vi "SimpleMotorFeedForward_Example_2.vi"() -> ()   [LabVIEW 2019]
uses:
  <vilib>/Rock Robotics/WPI/ThirdParty/JAS_Junk/TrajLib/LinearFilter_ResetToValue.vi
  <vilib>/Rock Robotics/WPI/ThirdParty/JAS_Junk/TrajLib/LinearFilter_Calculate.vi
  <vilib>/Rock Robotics/WPI/ThirdParty/JAS_Junk/TrajLib/SimpleMotorFF_Calculate.vi
  <vilib>/Rock Robotics/WPI/ThirdParty/JAS_Junk/TrajLib/LinearFilter_MovingAverage.vi
  <vilib>/Rock Robotics/WPI/ThirdParty/JAS_Junk/TrajLib/LinearFilter_LowPassBW1.vi
  <vilib>/Rock Robotics/WPI/ThirdParty/JAS_Junk/TrajLib/LinearFilter_LowPassBW2.vi
  <vilib>/Rock Robotics/WPI/ThirdParty/JAS_Junk/TrajLib/LinearFilter_HighPassBW1.vi
  <vilib>/Rock Robotics/WPI/ThirdParty/JAS_Junk/TrajLib/LinearFilter_HighPassBW2.vi
  <vilib>/Rock Robotics/WPI/ThirdParty/JAS_Junk/TrajLib/Trajectory_Library.lvlib
panel:
  in  "Tab Control":T1(tab)
  out "Running Ka AutoTune":bool
  in  "Execute Ka AutoTune":bool
  out "Filtered Setpoint \nRate of Change":dbl format="%11.3f"
  in  "Auto Setpoint":bool
  out "CO Trend":dbl(graph)
  out "SP, PV Trend":T2(graph)
  in  "Desired Speed":dbl(slide)=-0.22222222222222499 scale=-10.0..10.0 scale format="%#.1f"
  in  "Enable Noise":bool
  in  "Ks":dbl format="%#_13g"
  in  "Kv":dbl=0.1 format="%#_13g"
  in  "Ka":dbl format="%#_13g"
  out "Motor Dmd":dbl format="%13.3f"
  out "Filtered Speed":dbl format="%12.2f"
  out "Filtered Speed \nError":dbl format="%11.3f"
  in  "Ka Testing Parameters":T3={"Min SP"=0.0, "Max SP"=9.0, "Min Eval SP"=1.5, "Max Eval SP"=7.5, "Ramp Rate"=0.66}
  out "Test Complete":bool
  out "Ka Calc":dbl=-1.0 format="%#_8g"
  out "Ka StdDev":dbl=-1.0 format="%#_8g"
  out "Error":bool
  # "Simple Motor Feedforward Example 2"
  # "FT/SEC"
  # "FT/SEC"
  # "Sample procedure to tune Simple Motor Feedforward Ks, Kv, Ka.\n\nThis is just one possible method to do the tuning.  Other methods, including using the characterization tool, can be used.\n\n1) Set the Ka and Ks to 0.0.   Set Kv to be 1 / Estimated Maximum Speed.   (For many robots 10 feet/sec works as a starting point).\n     If using any closed loop control, such as a PID, disable the closed loop control, either by removing the code, or for the advanced\n    PID, putting it in manual mode.  (This simulation does not have a closed loop controller.)\n\n2)  Set the motor output at a small value.  (Example 0.15).  To do this set the speed demand to a small value, such as 1.5 Ft/Sec.\n      After the robot comes to constant speed, record the Motor Demand CO and Actual Speed (PV)\n\n3) Set the motor output to a large value (Example 0.90).   To do this, set the speed demand to a large value, such as 9.0 Ft/Sec\n     After the robot (or this simulation) comes to a constant speed, record the Motor Demand (CO) and the Actual Speed (PV).\n\n4) Ks and Kv can be calculated from the straight line equation:\n                               Motor Dmd CO = Sign( Speed_Setpoint) x Ks + Speed_Setpoint x Kv\n                                          Sign = 1 when Speed_Setoint > 0.0, \n                                          0 when Speed_Setpoint = 0 and, \n                                          -1 when Speed_Setpoint < 0\n\n5) The Ka term represents the additional Motor Demand CO needed to cancel the lag of the motor.   Technically, the Ka term\n      represents a \"lead\" function (sometimes referred to as a kicker circuit).  The amount that Ka adds to the Motor Demand CO\n      is  Ka x Speed_Setpoint Rate of Change (units/second).  Therefore, while the speed is ramping, one knows, or can be\n      calculated:   \n                             - Setpoint Rate of Change\n                             - Speed, speed setpoint, motor demand a time \"n\"\n                             - motor demand at time \"m\" where speed_m = speed_setpoint_n\n  \n    This should be enough data to calculate a value for Ka:\n                              Ka = (motor_demand_m - motor_demand_n ) / setpoint_rate_of_change\n\n     The Ka term will cause the speed to overshoot slightly during a ramp.  This is an expected side-affect of this type of \n     algorithm.  \n\n6) Test everything and look at the trend to ensure the response is acceptable.    Adjust as desired."
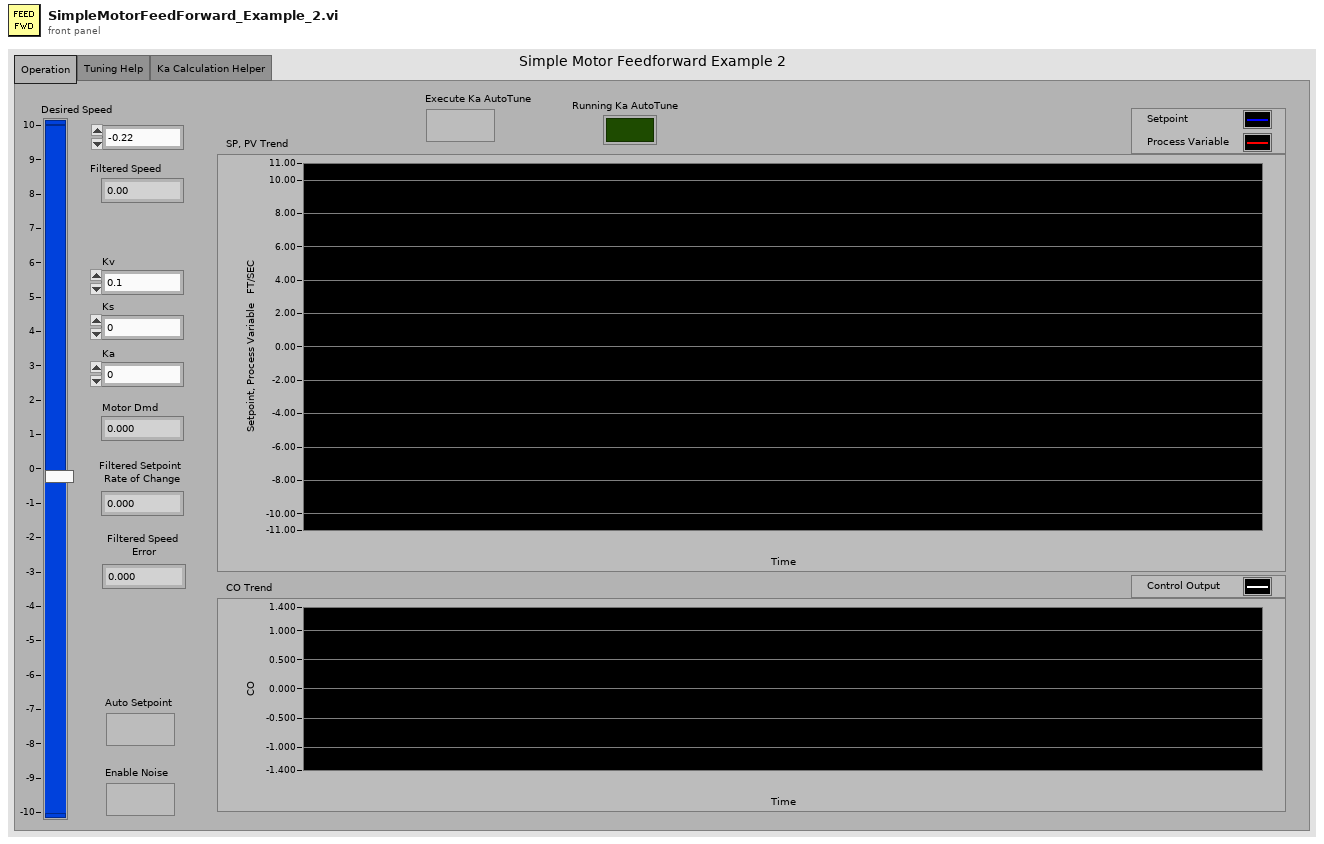
[diagram p1: front panel]
types:
  T1 = enum32{"Operation", "Tuning Help", "Ka Calculation Helper"}
  T2 = cluster{"SpeedSetpoint":dbl, "LeftWheelSpeed":dbl}
  T3 = cluster{"Min SP":dbl, "Max SP":dbl, "Min Eval SP":dbl, "Max Eval SP":dbl, "Ramp Rate":dbl}
  T4 = enum16{"Moving Average", "Low Pass 1st Order Butterworth", "Low Pass 2nd Order Butterworth", "High Pass 1st Order Butterworth", "High Pass 2nd Order Butterworth"}
  T5 = typedef "Trajectory_Library.lvlib/SIMPLE_MOTOR_FF.ctl" = cluster{"Ks":dbl, "Kv":dbl, "Ka":dbl, "KnInv":dbl}
  T6 = cluster{"Speed Setpoint Ft/Sec":dbl, "Motor Speed":dbl}
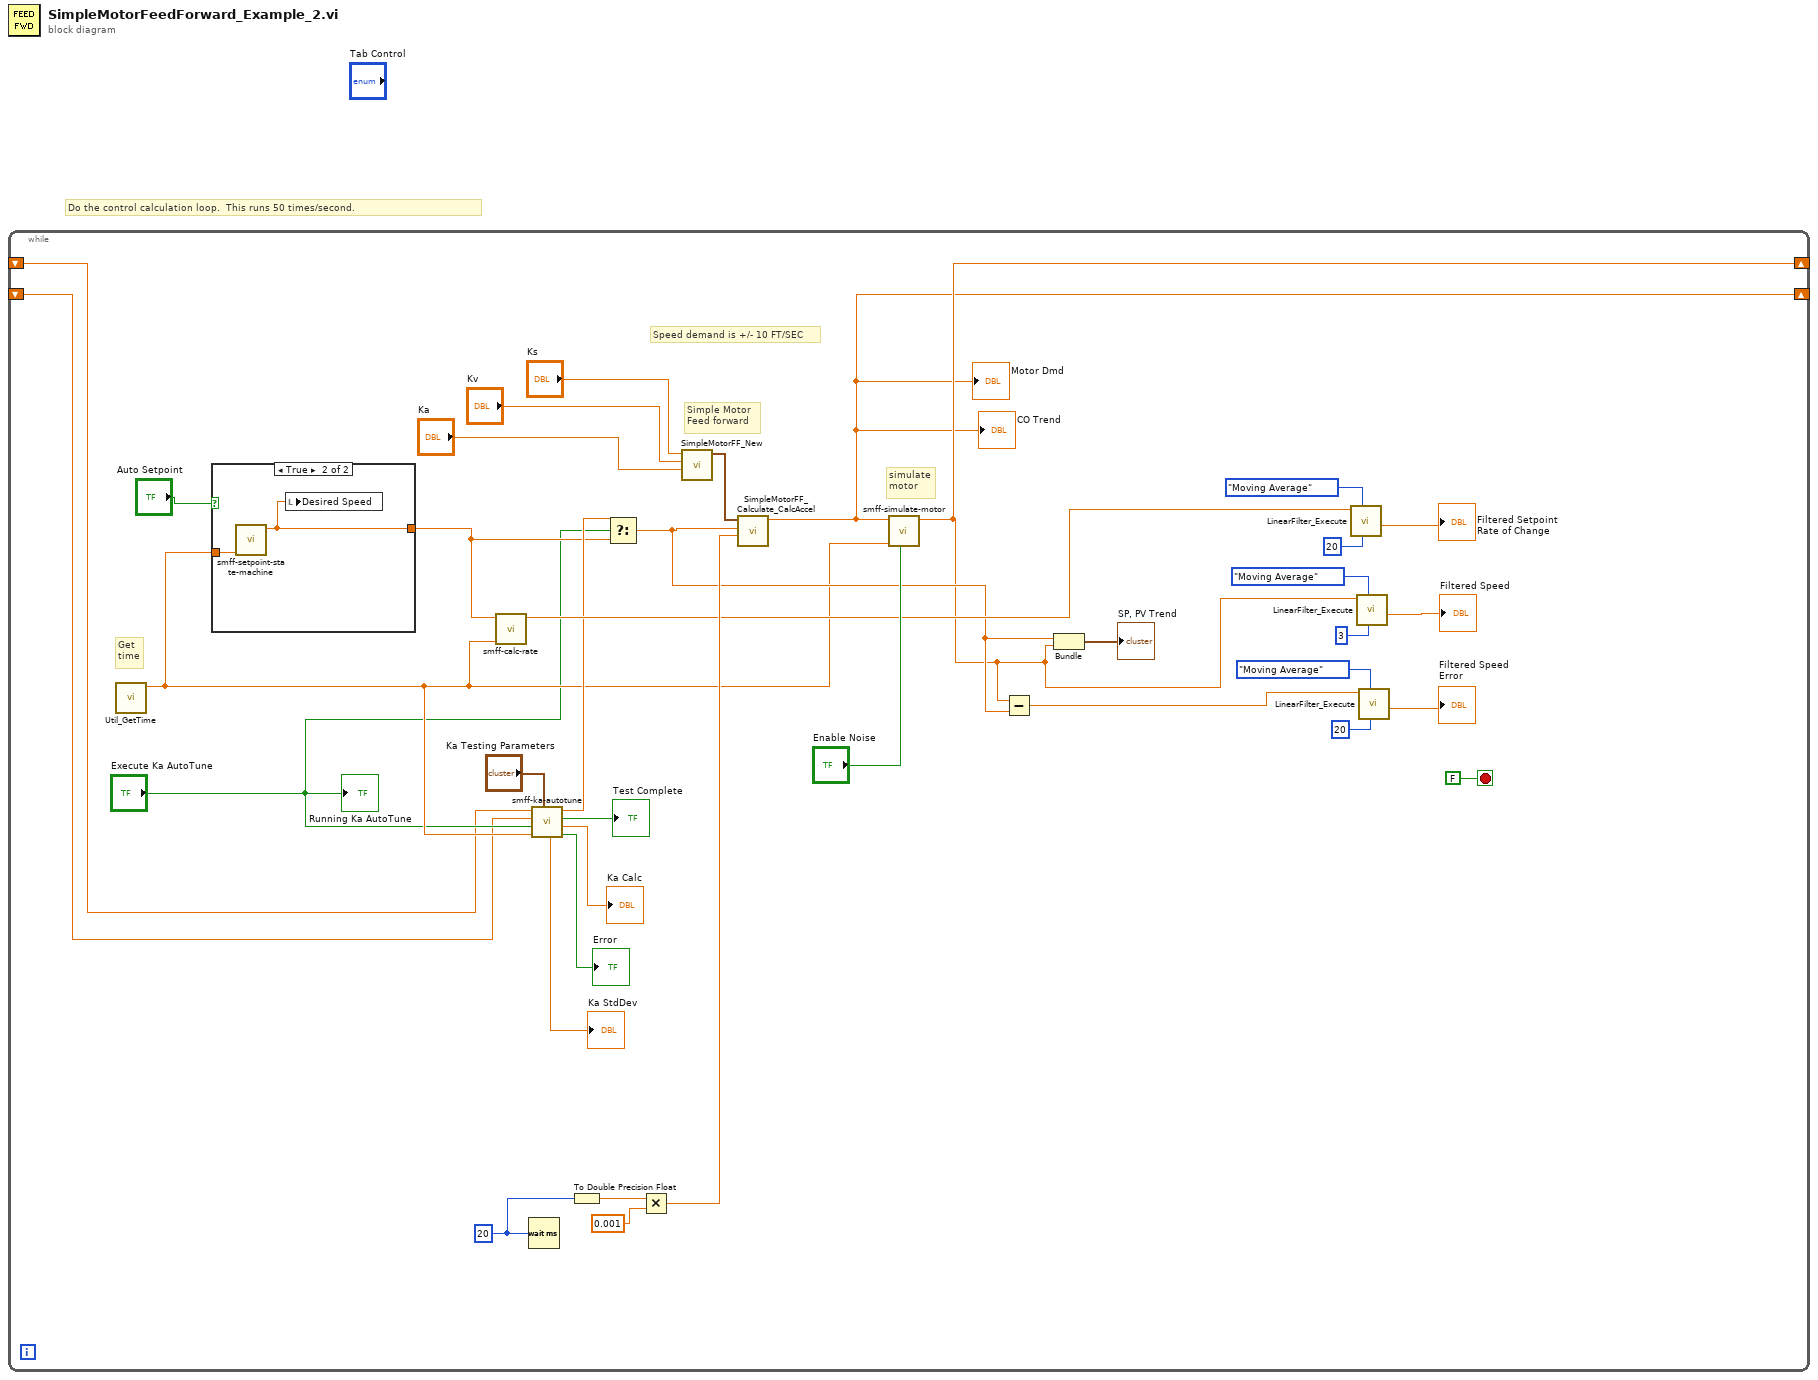
[diagram p0: block diagram]
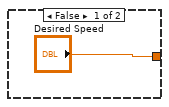
[diagram p2: hidden frame]
diagram:
  # "Do the control calculation loop.  This runs 50 times/second."
  n1 = while {
    shift-right: [w6] -> _
    shift-left: _ -> [w4]
    shift-right: [w5] -> _
    shift-left: _ -> [w3]
    stop <- FALSE stop-if-true
    w36 = u32 20 ("milliseconds to wait")
    # "Get\ntime"
    # "Speed demand is +/- 10 FT/SEC"
    # "simulate\nmotor"
    # "Simple Motor\nFeed forward"
    n2 = call <vilib>:"Util_GetTime.vi"() -> ("FPGA_Time_Seconds"=w8:dbl)  [unwired: 10 in, 1 out]
    n3 = case shown="True" "Auto Setpoint" {
      tunnel: w8 -> [_ w40]
      tunnel: ["Desired Speed" w39] -> w12
      frame False {
      }
      frame True {
        n4 = call "smff-setpoint-state-machine.vi"("Time pass through"=w40) -> ("Speed Setpoint Ft/Sec"=w39:dbl)  [unwired: 9 in, 1 out]
        n5 = local write "Desired Speed"(w39) -> ()
      }
    }
    n6 = call "smff-calc-rate.vi"("Time pass through"=w8, "Value"=w12) -> ("Value Rate"=w15:dbl)  [unwired: 9 in]
    n7 = Wait (ms)(milliseconds to wait=w36) -> ()  [unwired: 1 out]
    n8 = call "smff-ka-autotune.vi"("SimpleMotorFeedforward_KaTune_Pack"="Ka Testing Parameters", "PassThroughTime"=w8, "Run Test"="Execute Ka AutoTune", "ControlOutput CO"=w3, "ProcVariable PV"=w4) -> ("Error"=→"Error":bool, "Ka Calc"=→"Ka Calc":dbl, "Test Complete"=→"Test Complete":bool, "SetPoint"=w13:dbl, "Ka StdDev"=→"Ka StdDev":dbl)  [unwired: 2 out]
    n9 = To Double Precision Float(number=w36) -> (double precision float=w30:dbl)
    n10 = Select(t=w13, s="Execute Ka AutoTune", f=w12) -> (s? t:f=w14:dbl)
    n11 = Multiply(x=w30, y=0.001) -> (x*y=w28:dbl)
    n12 = call <vilib>:"SimpleMotorFF_New.vi"("Ka"="Ka", "Kv"="Kv", "Ks"="Ks") -> ("SIMPLE_MOTOR_FF"=w34:T5)  [unwired: 8 in]
    n13 = call <vilib>:"SimpleMotorFF_Calculate_CalcAccel.vi"("dT_Sec"=w28, "VelSp"=w14, "SIMPLE_MOTOR_FF"=w34) -> ("FeedForward"=w5:dbl)  [unwired: 8 in]
    "Motor Dmd" <- w5
    "CO Trend" <- w5
    n14 = call "smff-simulate-motor.vi"("Use Noise"="Enable Noise", "Time"=w8, "CO-ControlOutput"=w5) -> ("Motor Speed"=w6:dbl)  [unwired: 8 in]
    n15 = Subtract(x=w6, y=w14) -> (x-y=w26:dbl)
    n16 = Bundle("Speed Setpoint Ft/Sec"=w14, "Motor Speed"=w6) -> (→"SP, PV Trend":T6)  [unwired: 1 in]
    n17 = call <vilib>:"LinearFilter_Execute.vi"("Samples"=20, "Filter Type"=T4."Moving Average", "Input"=w15) -> ("Output"=→"Filtered Setpoint \nRate of Change":dbl)  [unwired: 7 in, 1 out]
    n18 = call <vilib>:"LinearFilter_Execute.vi"("Samples"=3, "Filter Type"=T4."Moving Average", "Input"=w6) -> ("Output"=→"Filtered Speed":dbl)  [unwired: 7 in, 1 out]
    n19 = call <vilib>:"LinearFilter_Execute.vi"("Samples"=20, "Filter Type"=T4."Moving Average", "Input"=w26) -> ("Output"=→"Filtered Speed \nError":dbl)  [unwired: 7 in, 1 out]
    "Running Ka AutoTune" <- "Execute Ka AutoTune"
  }
